vi "Version Constant.vi"(1 "SCC Revision when built":i32=137) -> (0 "Version":string="1.0.0.137")   [LabVIEW 2013]
doc: "Constant, Returns the version string"
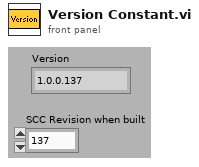
[diagram p1: front panel]
types:
  T1 = enum32{"invalid app kind", "Development System", "Run Time System", "Student Edition", "Embedded LabVIEW", "Evaluation", "Custom"}
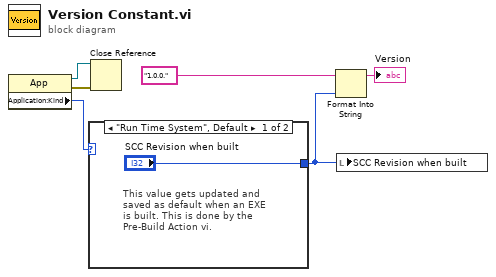
[diagram p0: block diagram]
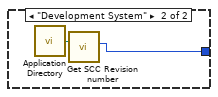
[diagram p2: hidden frame]
diagram:
  n1 = property class="App"() -> (reference out=w2:refnum<vi>, error out=w3:errorcluster, "Application:Kind"=w6:T1)  [unwired: 2 in]
  n2 = case shown="\"Run Time System\", Default" w6 {
    tunnel: ["SCC Revision when built" w8] -> w1
    frame "Run Time System", Default {
      # "This value gets updated and\nsaved as default when an EXE\nis built. This is done by the \nPre-Build Action vi."
    }
    frame "Development System" {
      n3 = call <vilib>:"Application Directory.vi"() -> ("Application Directory"=w9:path)
      n4 = call "Get SCC Revision number.vi"("path"=w9) -> ("Revision"=w8:i32)  [unwired: 10 in]
    }
  }
  n5 = Close Reference(reference=w2, error in (no error)=w3) -> ()  [unwired: 1 out]
  n6 = Format Into String(initial string="1.0.0." ("input 1"), w1) -> (resulting string=→"Version":string)  [unwired: 2 in, 1 out]
  n7 = local write "SCC Revision when built"(w1) -> ()
